vi "Create Events.vi"(7 "error in":errorcluster, 10 "Timer In":refnum<class "Timer.lvclass">) -> (0 "error out":errorcluster, 2 "Event Registration Refnum":refnum<event-registration>, 3 "Timer Out":refnum<class "Timer.lvclass">)   [LabVIEW 2021, in "Timer.lvclass"]
doc: "Creates the events required for the Worker's QMH's EHL."
uses:
  Timer.lvclass
  Timeout Settings.ctl
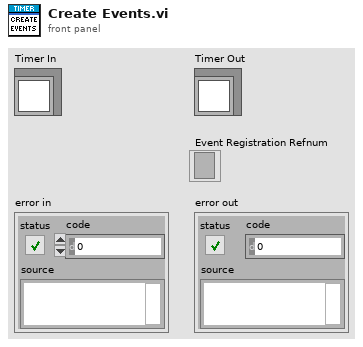
[diagram p1: front panel]
types:
  T1 = typedef "Timer.lvclass/Timeout Settings.ctl" = cluster{"Timeout (ms)":i32, "# Copies":i32}
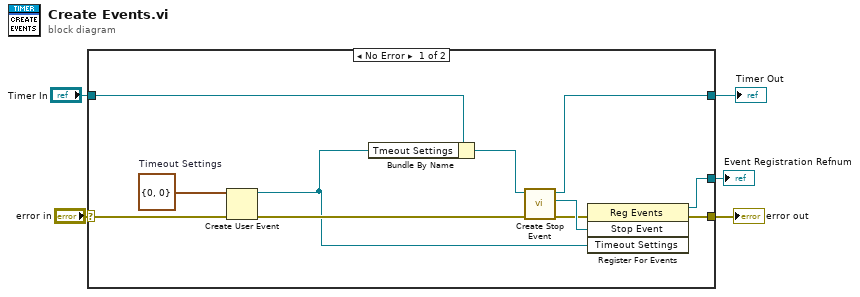
[diagram p0: block diagram]
diagram:
  n1 = case shown="No Error" "error in" {
    selector: "error in" -> [w9 w18]
    tunnel: [w16 w18] -> w5
    tunnel: [w15 _] -> w1
    tunnel: "Timer In" -> [w11 w17]
    tunnel: [w12 w17] -> w2
    frame No Error {
      w7 = T1 {"Timeout (ms)"=0, "# Copies"=0}  # Timeout Settings
      n2 = Create User Event(user event datatype=w7, error in=w9) -> (user event=w6:refnum<user-event>, error out=w8:errorcluster)
      n3 = Bundle By Name(cluster=w11, "Tmeout Settings"=w6) -> (w10:refnum<class "Timer.lvclass">)
      n4 = call-dynamic "Create Stop Event.vi"("error in"=w8, "Worker"=w10) -> ("error out"=w13:errorcluster, "Stop Event"=w14:refnum<user-event>, "Worker out"=w12:refnum<class "Timer.lvclass">)  [unwired: 7 in]
      n5 = register-events(error in=w13, w14, w6) -> (reference out=w15:refnum<event-registration>, error out=w16:errorcluster)  [unwired: 1 in]
    }
    frame Error {
    }
  }
  "error out" <- w5
  "Timer Out" <- w2
  "Event Registration Refnum" <- w1
